vi "GC EX Vacuum - Step 4.vi"(7 "Step":i32, 8 "error in":errorcluster, 9 "Test Results In":T8, 10 "Gas":T1, 11 "GC Configuration":T2) -> (0 "error out":errorcluster, 1 "Test Results Out":T8, 2 "Gas Out":T1 caption="Gas", 3 "GC Configuration Out":T2)   [LabVIEW 2015]
uses:
  Controls/Test Information.ctl
  Controls/Vacuum Test.ctl
  Controls/Test Timing.ctl
  Controls/Vaccum Thresholds.ctl
  Controls/Helium Test.ctl
  Controls/Helium Thresholds.ctl
  CAN Communication/Gas/Typedefs/Session Handle.ctl
  CAN Communication/Gas/Gas.lvclass
  Controls/Test Results.ctl
  Controls/Step Result.ctl
  CAN Communication/Gas/Typedefs/Valves.ctl
  SubVIs/Timing/Timing.lvlib
  User Interface/UI Handler/UI Handler.lvclass
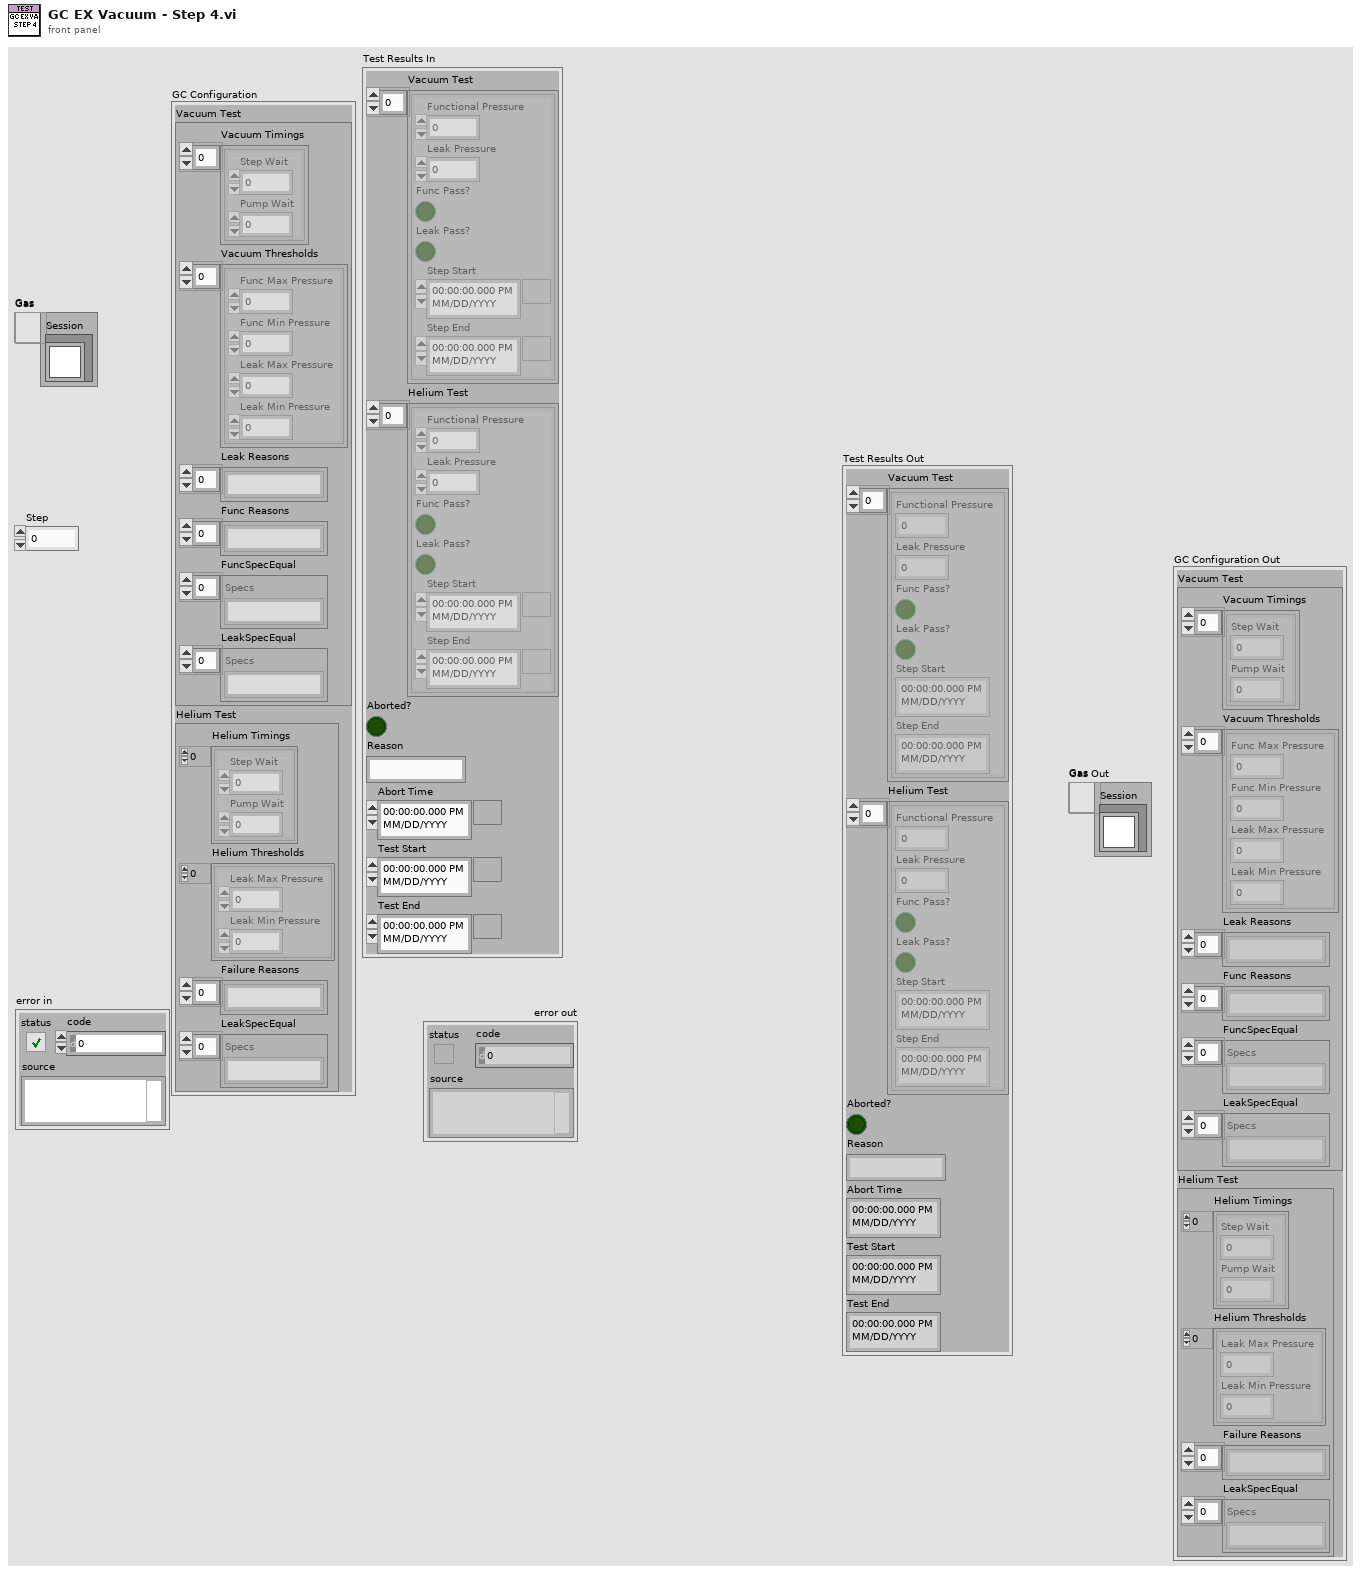
[diagram p1: front panel]
types:
  T1 = typedef "Gas.lvclass/Session Handle.ctl" = refnum<data-value>
  T2 = typedef "Test Information.ctl" = cluster{"Vacuum Test":T3, "Helium Test":T6}
  T3 = typedef "Vacuum Test.ctl" = cluster{"Vacuum Timings":T4[], "Vacuum Thresholds":T5[], "Leak Reasons":string[], "Func Reasons":string[], "FuncSpecEqual":string[], "LeakSpecEqual":string[]}
  T4 = typedef "Test Timing.ctl" = cluster{"Step Wait":dbl, "Pump Wait":dbl}
  T5 = typedef "Vaccum Thresholds.ctl" = cluster{"Func Max Pressure":dbl, "Func Min Pressure":dbl, "Leak Max Pressure":dbl, "Leak Min Pressure":dbl}
  T6 = typedef "Helium Test.ctl" = cluster{"Helium Timings":T4[], "Helium Thresholds":T7[], "Failure Reasons":string[], "LeakSpecEqual":string[]}
  T7 = typedef "Helium Thresholds.ctl" = cluster{"Leak Max Pressure":dbl, "Leak Min Pressure":dbl}
  T8 = typedef "Test Results.ctl" = cluster{"Vacuum Test":T9[], "Helium Test":T9[], "Aborted?":bool, "Reason":string, "Abort Time":timestamp, "Test Start":timestamp, "Test End":timestamp}
  T9 = typedef "Step Result.ctl" = cluster{"Functional Pressure":dbl, "Leak Pressure":dbl, "Func Pass?":bool, "Leak Pass?":bool, "Step Start":timestamp, "Step End":timestamp}
  T10 = typedef "Gas.lvclass/Valves.ctl" = u16
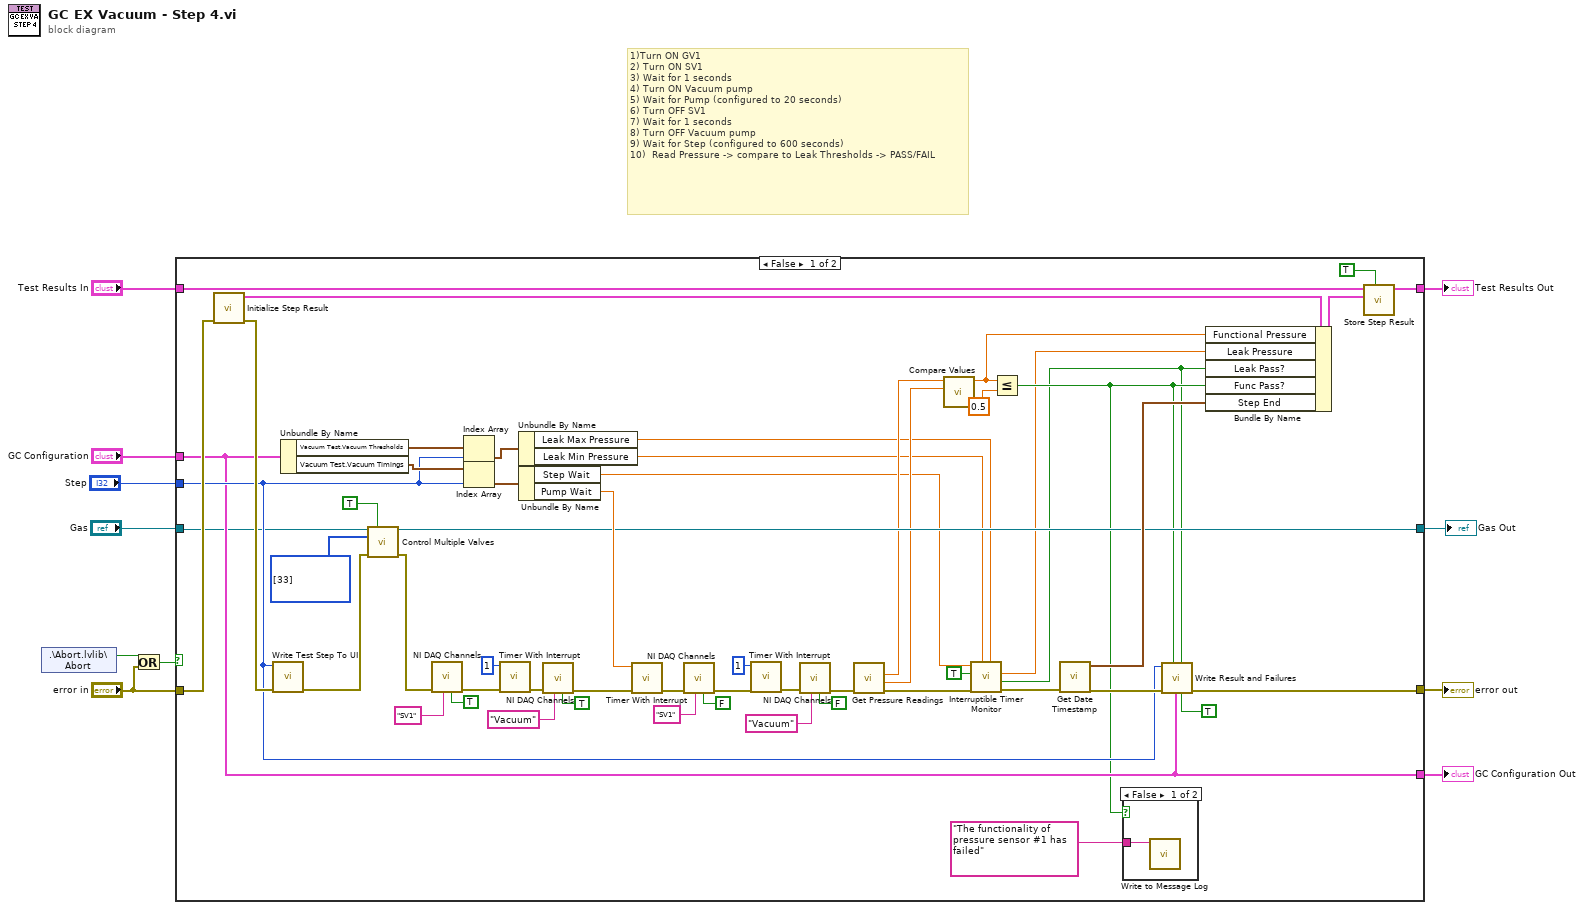
[diagram p0: block diagram]
diagram:
  # "1)Turn ON GV1\n2) Turn ON SV1\n3) Wait for 1 seconds\n4) Turn ON Vacuum pump\n5) Wait for Pump (configured to 20 seconds)\n6) Turn OFF SV1\n7) Wait for 1 seconds\n8) Turn OFF Vacuum pump\n9) Wait for Step (configured to 600 seconds)\n10)  Read Pressure -> compare to Leak Thresholds -> PASS/FAIL"
  n1 = shared-variable ".\\Abort.lvlib\\Abort"() -> (w10:bool)  [unwired: 1 in, 1 out]
  n2 = Or(x=w10, y="error in") -> (x .or. y?=w9:bool)
  n3 = case shown="False" w9 {
    tunnel: "error in" -> [w66 w70]
    tunnel: "Test Results In" -> [w63 w71]
    tunnel: [w64 w71] -> w7
    tunnel: [w54 w70] -> w6
    tunnel: "GC Configuration" -> [w52 w69]
    tunnel: "Step" -> [w53 _]
    tunnel: [w52 w69] -> w3
    tunnel: [w44 w68] -> w1
    tunnel: "Gas" -> [w48 w68]
    frame False {
      w47 = T10[] [33] items=["GV1"=33, "GV2"=34, "GV3"=35, "GV4"=36, "GV5"=37, "GV6"=38, "GV7"=39, "GV8"=40, "GV9"=41, "GV10"=42, "GV11"=43, "LV3"=51, "LV4"=52] ("Valves")
      n4 = call "Initialize Step Result.vi"("error in (no error)"=w66) -> ("error out"=w65:errorcluster, "New Step Result"=w62:T9)  [unwired: 8 in, 1 out]
      n5 = call "Write Test Step To UI.vi"("error in (no error)"=w65, "Step"=w53) -> ("error out"=w45:errorcluster)  [unwired: 9 in]
      n6 = Unbundle By Name(w52) -> ("Vacuum Test.Vacuum Thresholds"=w59:T5[], "Vacuum Test.Vacuum Timings"=w58:T4[])
      n7 = call "Control Multiple Valves.vi"("Session Handle in"=w48, "Energize?"=TRUE, "Valves"=w47, "error in (no error)"=w45) -> ("Session Handle out"=w44:T1, "error out"=w41:errorcluster)  [unwired: 8 in, 2 out]
      n8 = call "NI DAQ Channels.vi"("Control"=TRUE ("State"), "Channel"="SV1", "error in (no error)"=w41) -> ("error out"=w40:errorcluster)  [unwired: 7 in, 1 out]
      n9 = Index Array(array=w59, index=w53) -> (element=w56:T5)
      n10 = Index Array(array=w58, index=w53) -> (element=w57:T4)
      n11 = call "Timer With Interrupt.vi"("error in (no error)"=w40, "Wait (s)"=1) -> ("error out"=w38:errorcluster)  [unwired: 7 in, 2 out]
      n12 = Unbundle By Name(w56) -> ("Leak Max Pressure"=w18:dbl, "Leak Min Pressure"=w19:dbl)
      n13 = Unbundle By Name(w57) -> ("Step Wait"=w21:dbl, "Pump Wait"=w50:dbl)
      n14 = call "NI DAQ Channels.vi"("Control"=TRUE ("State"), "Channel"="Vacuum", "error in (no error)"=w38) -> ("error out"=w37:errorcluster)  [unwired: 7 in, 1 out]
      n15 = call "Timer With Interrupt.vi"("error in (no error)"=w37, "Wait (s)"=w50) -> ("error out"=w35:errorcluster)  [unwired: 7 in, 2 out]
      n16 = call "NI DAQ Channels.vi"("Control"=FALSE ("State"), "Channel"="SV1", "error in (no error)"=w35) -> ("error out"=w34:errorcluster)  [unwired: 7 in, 1 out]
      n17 = call "Timer With Interrupt.vi"("error in (no error)"=w34, "Wait (s)"=1) -> ("error out"=w32:errorcluster)  [unwired: 7 in, 2 out]
      n18 = call "NI DAQ Channels.vi"("Control"=FALSE ("State"), "Channel"="Vacuum", "error in (no error)"=w32) -> ("error out"=w31:errorcluster)  [unwired: 7 in, 1 out]
      n19 = call "Get Pressure Readings.vi"("error in (no error)"=w31) -> ("error out"=w23:errorcluster, "GAS Pressure 2"=w28:dbl, "GAS Pressure 1"=w29:dbl)  [unwired: 6 in, 2 out]
      n20 = call "Compare Values.vi"("P2"=w28, "P1"=w29) -> ("Abs Diff"=w27:dbl)  [unwired: 9 in]
      n21 = call "Interruptible Timer Monitor.vi"("Max"=w18, "Min"=w19, "error in (no error)"=w23, "Update UI?"=TRUE, "Wait (s)"=w21) -> ("error out"=w22:errorcluster, "In Range?"=w16:bool, "Leak Rate"=w17:dbl)  [unwired: 2 in, 2 out]
      n22 = Less Or Equal?(x=w27, y=0.5) -> (x <= y?=w25:bool)
      n23 = call "Get Date Timestamp.vi"("error in (no error)"=w22) -> ("error out"=w55:errorcluster, "current time"=w60:timestamp)  [unwired: 9 in]
      n24 = case shown="False" w25 {
        tunnel: "The functionality of pressure sensor #1 has failed" ("Message") -> [w67 _]
        frame False {
          n25 = call "Write to Message Log.vi"("Message"=w67) -> ()  [unwired: 10 in, 1 out]
        }
        frame True {
        }
      }
      n26 = call "Write Result and Failures.vi"("Vacuum?"=TRUE, "Leak"=w16, "GC Configuration"=w52, "Func"=w25, "error in (no error)"=w55, "Step"=w53) -> ("error out"=w54:errorcluster)  [unwired: 5 in]
      n27 = Bundle By Name(cluster=w62, "Functional Pressure"=w27, "Leak Pressure"=w17, "Leak Pass?"=w16, "Func Pass?"=w25, "Step End"=w60) -> (w61:T9)
      n28 = call "Store Step Result.vi"("Vacuum?"=TRUE, "Step Result"=w61, "Test Results In"=w63) -> ("Test Results Out"=w64:T8)  [unwired: 8 in]
    }
    frame True {
    }
  }
  "error out" <- w6
  "Test Results Out" <- w7
  "GC Configuration Out" <- w3
  "Gas Out" <- w1
